vi "ActorDatabase-PerformDelete.vi"(7 "Payload From Actor":string, 8 "error in (no error)":errorcluster, 11 "Database-Actor in":refnum<class "PartCertDatabase-Actor.lvclass">) -> (0 "error out":errorcluster, 3 "Database-Actor out":refnum<class "PartCertDatabase-Actor.lvclass">)   [LabVIEW 2013, in "PartCertDatabase-Actor.lvclass"]
uses:
  PartCertDatabase-Actor.lvclass
  PartCertDatabase-Actor.lvclass/PartCertDatabase-Actor.ctl
  Reuse Library/Database API/PartCertDatabase-API.lvclass
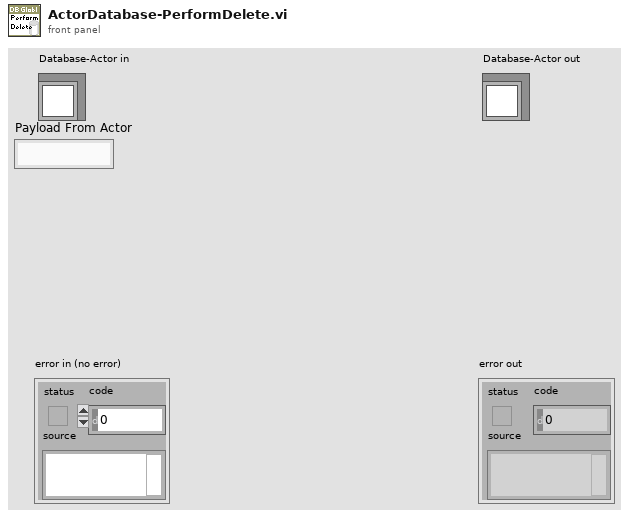
[diagram p1: front panel]
types:
  T1 = cluster{"Table":string, "SQL Statement":string, "Update All":bool, "Payload":string, "Reply Command":string, "Type Of Insertion":i32}
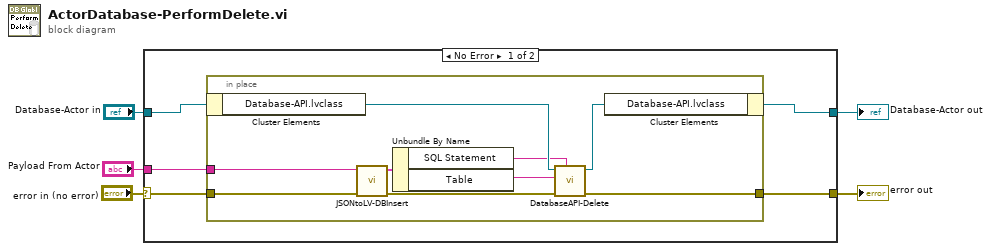
[diagram p0: block diagram]
diagram:
  n1 = case shown="No Error" "error in (no error)" {
    selector: "error in (no error)" -> [w10 w21]
    tunnel: [w9 w21] -> w4
    tunnel: [w7 w20] -> w2
    tunnel: "Database-Actor in" -> [w8 w20]
    tunnel: "Payload From Actor" -> [w6 _]
    frame No Error {
      n2 = in-place {
        in-place-border: w10 -> [w13]
        in-place-border: [w12] -> w9
        in-place-border: w6 -> [w11]
        n3 = in-place-cluster #1(w8) -> ("Database-API.lvclass"=w19:refnum<class "PartCertDatabase-API.lvclass">)
        n4 = call "JSONtoLV-DBInsert.vi"("error in"=w13, "Output JSON Object"=w11) -> ("error out"=w14:errorcluster, "value"=w17:T1)  [unwired: 8 in]
        n5 = Unbundle By Name(w17) -> ("SQL Statement"=w15:string, "Table"=w16:string)
        n6 = call "DatabaseAPI-Delete.vi"("Where Statement"=w15, "error in (no error)"=w14, "table"=w16, "Database-API in"=w19) -> ("error out"=w12:errorcluster, "Database-API out"=w18:refnum<class "PartCertDatabase-API.lvclass">)  [unwired: 6 in]
        n7 = in-place-cluster #1("Database-API.lvclass"=w18) -> (w7:refnum<class "PartCertDatabase-Actor.lvclass">)
      }
    }
    frame Error {
    }
  }
  "error out" <- w4
  "Database-Actor out" <- w2
